vi "Initialise Music.vi"(8 "error in (no error)":errorcluster, 11 "Main Controller Actor in":refnum<class "Main Controller Actor.lvclass">) -> (0 "error out":errorcluster, 3 "Main Controller Actor out":refnum<class "Main Controller Actor.lvclass">)   [LabVIEW 2021, in "Main Controller Actor.lvclass"]
uses:
  Main Controller Actor.lvclass
  Main Controller Actor.lvclass/Main Controller Actor.ctl
  LabBASSMOD2/LabBASSMOD2.lvlib
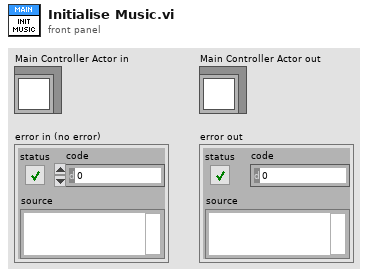
[diagram p1: front panel]
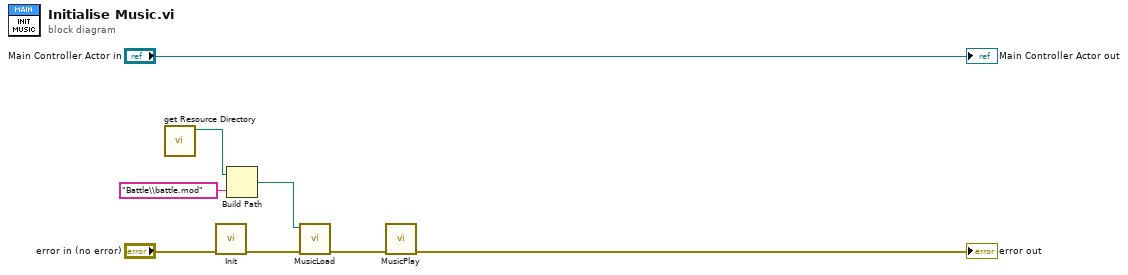
[diagram p0: block diagram]
diagram:
  n1 = call "get Resource Directory.vi"() -> ("Resource Directory"=w4:path)  [unwired: 11 in]
  n2 = call "Init.vi"("error in (no error)"="error in (no error)") -> ("error out"=w2:errorcluster)  [unwired: 9 in, 1 out]
  n3 = Build Path(base path=w4, name or relative path="Battle\\battle.mod") -> (appended path=w5:path)
  n4 = call "MusicLoad.vi"("error in (no error)"=w2, "path"=w5) -> ("error out"=w6:errorcluster)  [unwired: 9 in]
  n5 = call "MusicPlay.vi"("error in (no error)"=w6) -> ("error out"=→"error out":errorcluster)  [unwired: 10 in]
  "Main Controller Actor out" <- "Main Controller Actor in"
